vi "Apply rules.vi"(5 "All References":refnum<vi>[](array[refnum]), 6 "Error in":errorcluster, 7 "Relevant control names":string[](array[string]), 8 "Relevant controls":refnum<vi>[](array[refnum]), 9 "Rules to apply":T1[](array[typedef])) -> (0 "Error out":errorcluster)   [LabVIEW 2019, in "LSS.lvlib"]
doc: "Evaluate the criteria passed in and apply the resulting effects if the criteria have been met.\n\n<b>Inputs:</b>\n<b>Rules to apply</b> - For the event just generated, this is the list of critera to check.\n<b>All References</b> - List of every front panel object that can be stylized using LSS.\n<b>Relevant controls</b> - List of controls that have registered events. These are the ones the criteria will sort through to check for validity.\n<b>Relevant control names</b> - Used as the reference point for the criteria to pull out the correct control reference.\n<b>Error In</b> - Standard Error In terminal.\n\n<b>Outputs:</b>\n<b>Error Out</b> - Standard Error out terminal."
uses:
  LSS.lvlib
  Controls/Rule.ctl
  Controls/Criteria.ctl
  Controls/Comparison Types.ctl
  Controls/Effects.ctl
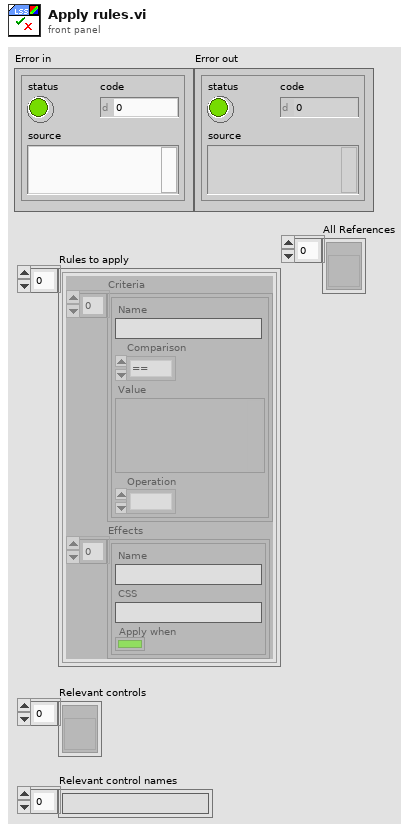
[diagram p1: front panel]
types:
  T1 = typedef "LSS.lvlib/Rule.ctl" = cluster{"Criteria":T2[], "Effects":T4[]}
  T2 = typedef "LSS.lvlib/Criteria.ctl" = cluster{"Name":string, "Comparison":T3, "Value":variant, "Operation":enum16{"Stack", "&&", "||"}}
  T3 = typedef "LSS.lvlib/Comparison Types.ctl" = enum16{"==", "!=", "<", ">", "<=", ">="}
  T4 = typedef "LSS.lvlib/Effects.ctl" = cluster{"Name":string, "CSS":string, "Apply when":bool}
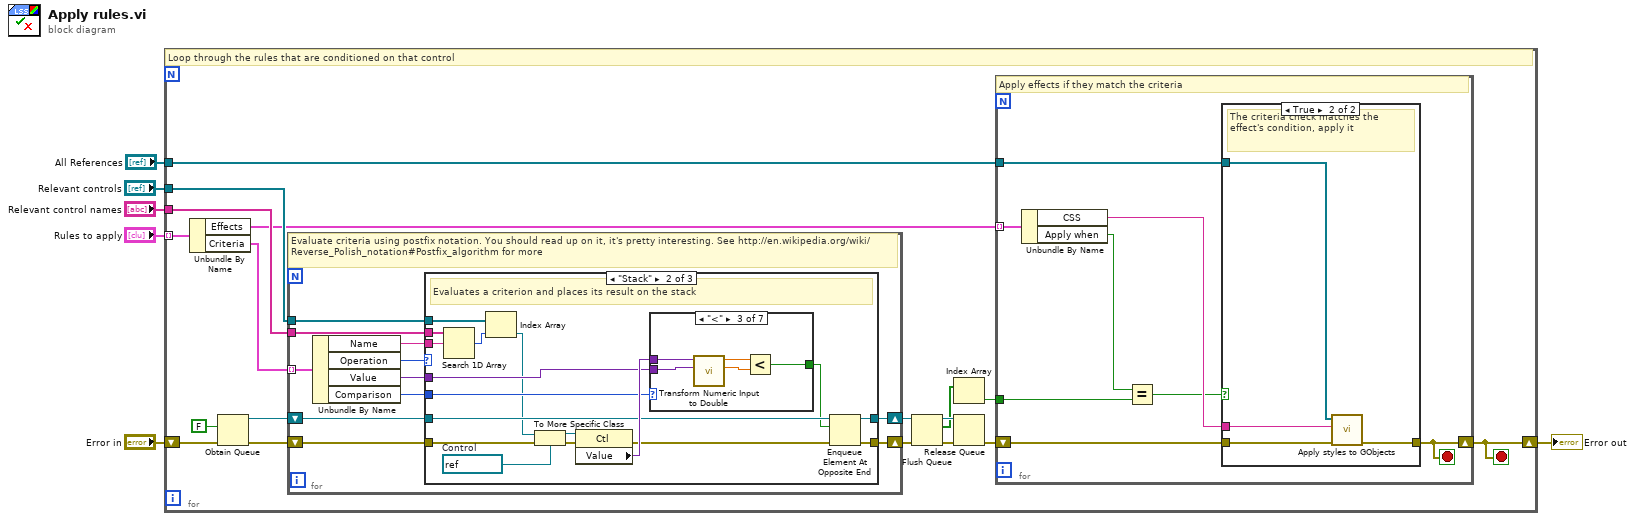
[diagram p0: block diagram]
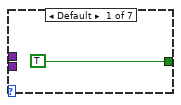
[diagram p4: hidden frame]
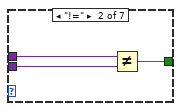
[diagram p5: hidden frame]
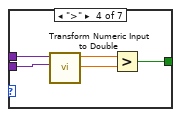
[diagram p6: hidden frame]
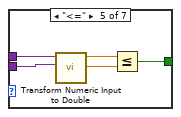
[diagram p7: hidden frame]
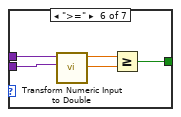
[diagram p8: hidden frame]
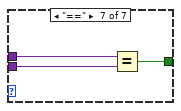
[diagram p9: hidden frame]
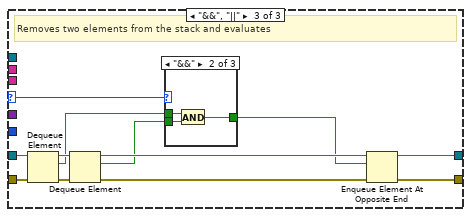
[diagram p10: hidden frame]
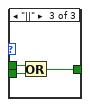
[diagram p12: hidden frame]
diagram:
  n1 = for {
    tunnel: "Rules to apply" -> [w24] mode=indexing
    tunnel: "Relevant control names" -> [w21]
    tunnel: "Relevant controls" -> [w22]
    shift-right: [w7] -> w2
    shift-left: "Error in" -> [w11]
    tunnel: "All References" -> [w8]
    stop <- w7 stop-if-true
    # "Loop through the rules that are conditioned on that control"
    n2 = Unbundle By Name(w24) -> ("Effects"=w9:T4[], "Criteria"=w23:T2[])
    n3 = Obtain Queue(element data type=FALSE, error in (no error)=w11) -> (queue out=w16:refnum<queue>, error out=w10:errorcluster)  [unwired: 3 in, 1 out]
    n4 = for {
      tunnel: w23 -> [w44] mode=indexing
      tunnel: w21 -> [w48]
      tunnel: w22 -> [w47]
      shift-right: [w45] -> w13
      shift-left: w10 -> [w46]
      shift-right: [w41] -> w17
      shift-left: w16 -> [w40]
      # "Evaluate criteria using postfix notation. You should read up on it, it's pretty interesting. See http://en.wikipedia.org/wiki/Reverse_Polish_notation#Postfix_algorithm for more"
      n5 = Unbundle By Name(w44) -> ("Name"=w42:string, "Operation"=w39:enum16{"Stack", "&&", "||"}, "Value"=w43:variant, "Comparison"=w38:T3)
      n6 = case shown="\"Stack\"" w39 {
        selector: w39 -> [_ _ w101]
        tunnel: w48 -> [_ w67 _]
        tunnel: w47 -> [_ w66 _]
        tunnel: w46 -> [w49 w52 w96]
        tunnel: [w49 w56 w95] -> w45
        tunnel: w43 -> [_ w63 _]
        tunnel: w38 -> [_ w62 _]
        tunnel: w42 -> [_ w61 _]
        tunnel: w40 -> [w50 w60 w102]
        tunnel: [w50 w58 w97] -> w41
        frame Default {
          # "No operation"
        }
        frame "Stack" {
          w53 = refnum<vi> refnum  # Control
          # "Evaluates a criterion and places its result on the stack"
          n7 = Search 1D Array(1D array=w67, element=w61) -> (index of element=w65:i32)  [unwired: 1 in]
          n8 = Index Array(array=w66, index=w65) -> (element=w54:refnum<vi>)
          n9 = To More Specific Class(target class=w53, reference=w54, error in=w52) -> (specific class reference=w55:refnum<vi>, error out=w51:errorcluster)
          n10 = property class="Ctl"(reference=w55, error in=w51) -> (error out=w57:errorcluster, "Value"=w64:variant)  [unwired: 1 out]
          n11 = case shown="\"<\"" w62 {
            tunnel: w64 -> [_ w71 w76 w80 w85 w90 w94]
            tunnel: [TRUE w70 w75 w81 w86 w91 w92] -> w59
            tunnel: w63 -> [_ w69 w74 w79 w84 w89 w93]
            frame Default {
            }
            frame "!=" {
              n12 = Not Equal?(x=w71, y=w69) -> (x != y?=w70:bool)
            }
            frame "<" {
              n13 = call "Transform Numeric Input to Double.vi"("LSS String Value as Variant"=w74, "Value from Control"=w76) -> ("Expected"=w73:dbl, "Control"=w72:dbl)  [unwired: 8 in]
              n14 = Less?(x=w72, y=w73) -> (x < y?=w75:bool)
            }
            frame ">" {
              n15 = call "Transform Numeric Input to Double.vi"("LSS String Value as Variant"=w79, "Value from Control"=w80) -> ("Expected"=w77:dbl, "Control"=w78:dbl)  [unwired: 8 in]
              n16 = Greater?(x=w78, y=w77) -> (0:w81:bool)
            }
            frame "<=" {
              n17 = call "Transform Numeric Input to Double.vi"("LSS String Value as Variant"=w84, "Value from Control"=w85) -> ("Expected"=w82:dbl, "Control"=w83:dbl)  [unwired: 8 in]
              n18 = Less Or Equal?(x=w83, y=w82) -> (x <= y?=w86:bool)
            }
            frame ">=" {
              n19 = call "Transform Numeric Input to Double.vi"("LSS String Value as Variant"=w89, "Value from Control"=w90) -> ("Expected"=w87:dbl, "Control"=w88:dbl)  [unwired: 8 in]
              n20 = Greater Or Equal?(x=w88, y=w87) -> (x >= y?=w91:bool)
            }
            frame "==" {
              n21 = Equal?(x=w94, y=w93) -> (x = y?=w92:bool)
            }
          }
          n22 = Enqueue Element At Opposite End(queue=w60, element=w59, error in (no error)=w57) -> (queue out=w58:refnum<queue>, error out=w56:errorcluster)  [unwired: 1 in, 1 out]
        }
        frame "&&", "||" {
          # "Removes two elements from the stack and evaluates"
          n23 = Dequeue Element(queue=w102, error in (no error)=w96) -> (queue out=w103:refnum<queue>, element=w99:bool, error out=w104:errorcluster)  [unwired: 1 in, 1 out]
          n24 = Dequeue Element(queue=w103, error in (no error)=w104) -> (queue out=w105:refnum<queue>, element=w100:bool, error out=w106:errorcluster)  [unwired: 1 in, 1 out]
          n25 = case shown="\"&&\"" w101 {
            tunnel: w100 -> [_ w109 w112]
            tunnel: w99 -> [w107 w110 w113]
            tunnel: [w107 w108 w111] -> w98
            frame Default {
            }
            frame "&&" {
              n26 = And(x=w110, y=w109) -> (x .and. y?=w108:bool)
            }
            frame "||" {
              n27 = Or(x=w113, y=w112) -> (x .or. y?=w111:bool)
            }
          }
          n28 = Enqueue Element At Opposite End(queue=w105, element=w98, error in (no error)=w106) -> (queue out=w97:refnum<queue>, error out=w95:errorcluster)  [unwired: 1 in, 1 out]
        }
      }
    }
    n29 = Flush Queue(queue=w17, error in (no error)=w13) -> (queue out=w18:refnum<queue>, remaining elements=w15:bool[], error out=w19:errorcluster)
    n30 = Index Array(array=w15) -> (element=w14:bool)  [unwired: 1 in]
    n31 = Release Queue(queue=w18, error in (no error)=w19) -> (error out=w12:errorcluster)  [unwired: 1 in, 2 out]
    n32 = for {
      tunnel: w9 -> [w32] mode=indexing
      tunnel: w8 -> [w31]
      tunnel: w14 -> [w30]
      shift-right: [w25] -> w7
      shift-left: w12 -> [w29]
      stop <- w25 stop-if-true
      # "Apply effects if they match the criteria"
      n33 = Unbundle By Name(w32) -> ("CSS"=w28:string, "Apply when"=w27:bool)
      n34 = Equal?(x=w27, y=w30) -> (x = y?=w26:bool)
      n35 = case shown="True" w26 {
        tunnel: w28 -> [_ w34]
        tunnel: w29 -> [w33 w37]
        tunnel: [w33 w36] -> w25
        tunnel: w31 -> [_ w35]
        frame False {
          # "The criteria check didn't match the effect's condition, noop"
        }
        frame True {
          # "The criteria check matches the effect's condition, apply it"
          n36 = call "Apply styles to GObjects.vi"("Error In"=w37, "Style Sheet"=w34, "Front Panel Objects"=w35) -> ("Error Out"=w36:errorcluster)  [unwired: 7 in, 1 out]
        }
      }
    }
  }
  "Error out" <- w2
